vi "Destroy.vi"(8 "error in (no error)":errorcluster, 11 "Dispatcher Interface in":refnum<class "Dispatcher Interface.lvclass">) -> (0 "error out":errorcluster)   [LabVIEW 2017, in "DSF Core.lvlib" / "Dispatcher Interface.lvclass"]
uses:
  Dispatcher Interface.lvclass
  C:/Users/Admin/Desktop/Data Sharing Framework/Source/Core/Engine/Classes/Interfaces/Interface/Interface.lvclass
  Interface/Interface.lvclass
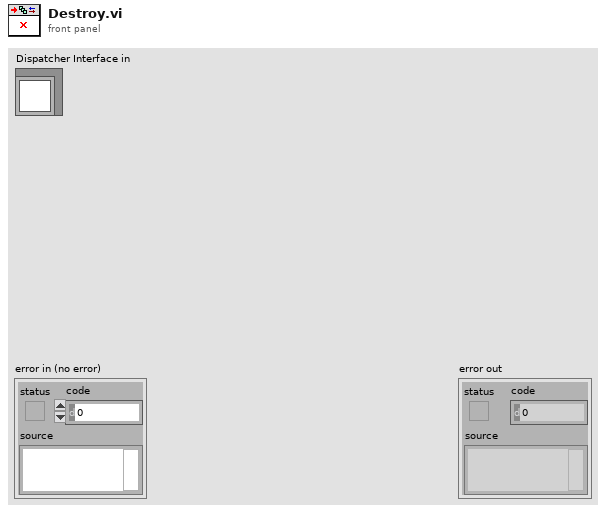
[diagram p1: front panel]
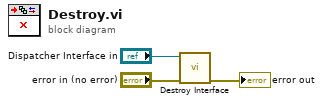
[diagram p0: block diagram]
diagram:
  n1 = call "Destroy Interface.vi"("error in (no error)"="error in (no error)", "Interface in"="Dispatcher Interface in") -> ("error out"=→"error out":errorcluster)  [unwired: 7 in, 2 out]
